vi "Change Boolean Image.vi"(6 "Mouse Position":T1, 7 "User VI Ref":refnum<vi>, 8 "Is Multi-select?":bool, 9 "Remaining Items":refnum<vi>[](array[refnum]), 10 "Affected Items":cluster{"Controls":refnum<vi>[]}, 11 "Menu Refnum":refnum<k9>) -> (3 "Menu Items To Add":T2[](array[typedef]))   [LabVIEW 2021]
doc: "This implementation of the right click menu VI will set the \"Boolean Type\" for a given Boolean control(s) for a VI. It will categorize the type of the button that is being used so that Theme-ing can be applied appropriately.\n\n<b>Original</b>: This VI is part of a plug-in for modifying the LabVIEW shortcut menus. This is the builder VI which is called when the shortcut menu is built. It tells LabVIEW which shortcut menu items to add to the menu."
uses:
  <resource>/plugins/PopupMenus/support/Shortcut Menu Item Definition.ctl
  <resource>/plugins/PopupMenus/support/Transaction Control.ctl
  <resource>/plugins/PopupMenus/support/Position In Menu.ctl
  <resource>/plugins/PopupMenus/support/Relative Position.ctl
  <resource>/plugins/PopupMenus/support/Checkmark Status.ctl
  <resource>/plugins/PopupMenus/support/Enabled Menu Item Status.ctl
  <vilib>/Utility/miscctls.llb/LVPositionTypeDef.ctl
panel:
  # "Rules a popup plug-in must follow:\n* This VI's file name must match the file name of the LLB -- only the file extensions should be different.\n* This VI must have debugging disabled or it will be ignored as a plug-in.\n* For all menu items, \"tag suffix + file name of this VI\" must be less than 240 characters.\n* You can disconnect the \"Affected Items\" from the typedef to make the plug-in load faster. The typedef is only there to assist you in keeping this VI and the execution VI using to the same type.\n* All controls on this panel except \"Affected Items\" are locked to prevent accidental edits. Do not change the types or the names of controls other than the elements inside the \"Affected Items\" cluster.\n* See Context Help for more information on the individual controls."
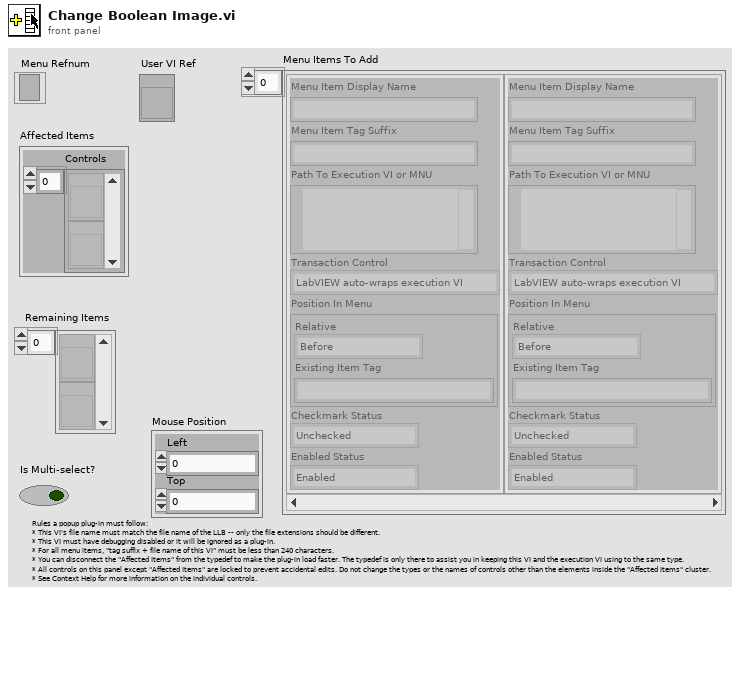
[diagram p1: front panel]
types:
  T1 = typedef "LVPositionTypeDef.ctl" = cluster{"Left":i32, "Top":i32}
  T2 = typedef "Shortcut Menu Item Definition.ctl" = cluster{"Menu Item Display Name":string, "Menu Item Tag Suffix":string, "Path To Execution VI or MNU":path, "Transaction Control":T3, "Position In Menu":T4, "Checkmark Status":T6, "Enabled Status":T7}
  T3 = typedef "Transaction Control.ctl" = enum8{"LabVIEW auto-wraps execution VI", "Execution VI will define if needed"}
  T4 = typedef "Position In Menu.ctl" = cluster{"Relative":T5, "Existing Item Tag":string}
  T5 = typedef "Relative Position.ctl" = enum8{"Before", "Instead of", "After", "Into Submenu"}
  T6 = typedef "Checkmark Status.ctl" = enum8{"Unchecked", "Checked"}
  T7 = typedef "Enabled Menu Item Status.ctl" = enum8{"Enabled", "Disabled"}
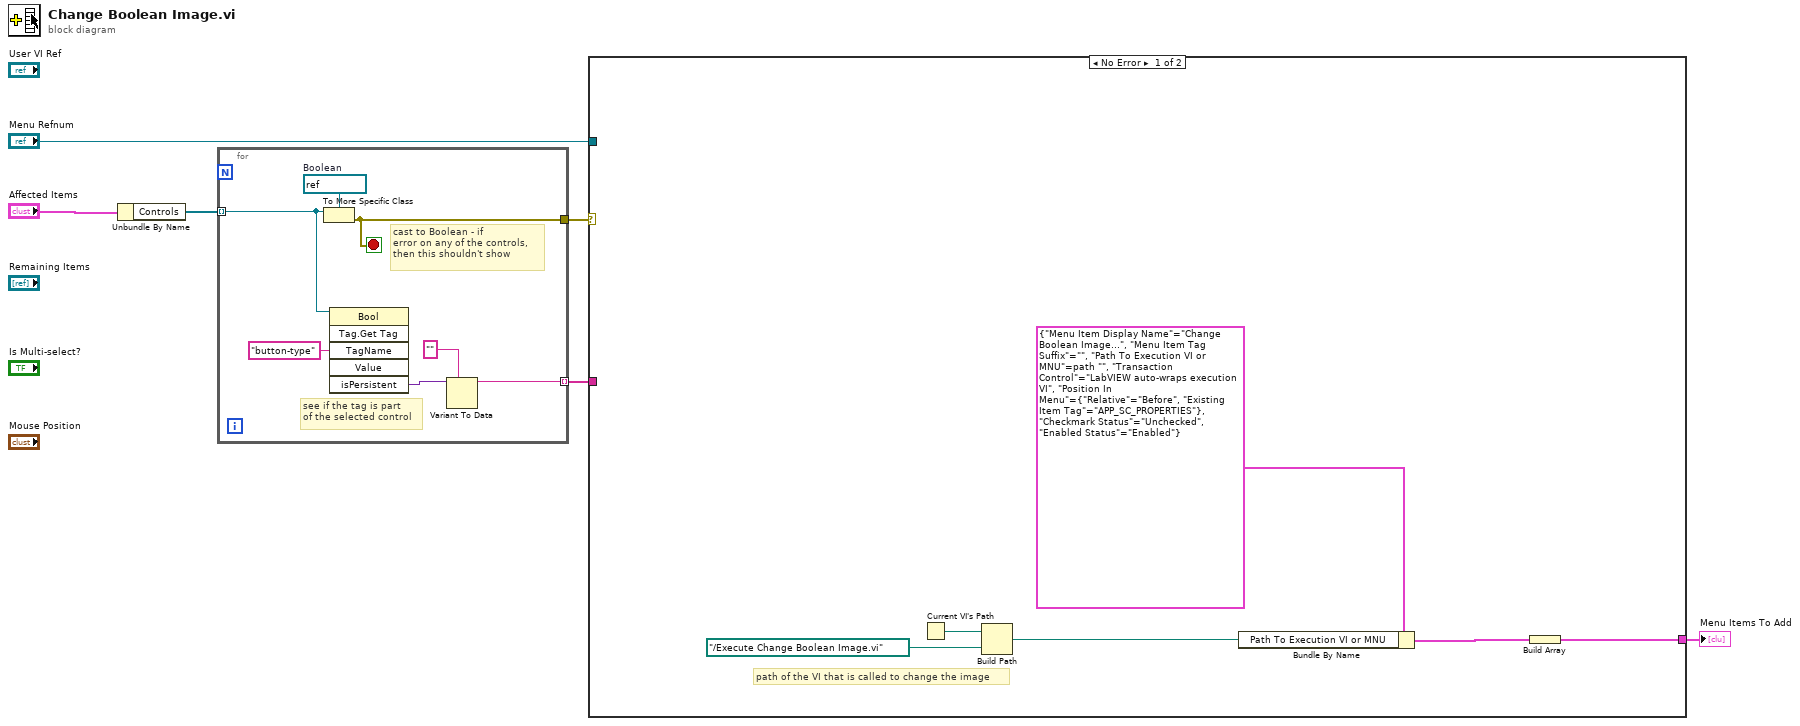
[diagram p0: block diagram]
diagram:
  n1 = Unbundle By Name("Affected Items") -> ("Controls"=w4:refnum<vi>[])
  n2 = for {
    tunnel: w4 -> [w7] mode=indexing
    tunnel: [w12] -> w3
    tunnel: [w8] -> w1 mode=indexing
    stop <- w12 stop-if-true
    w13 = refnum<vi> refnum  # Boolean
    # "cast to Boolean - if\nerror on any of the controls, \nthen this shouldn't show"
    # "see if the tag is part \nof the selected control"
    n3 = To More Specific Class(target class=w13, reference=w7) -> (error out=w12:errorcluster)  [unwired: 1 in, 1 out]
    n4 = invoke class="Bool" method="Tag.Get Tag"(reference=w7, "TagName"="button-type" ("Tag Name")) -> ("isPersistent"=w10:variant)  [unwired: 4 in, 5 out]
    n5 = Variant To Data(type="", Variant=w10) -> (data=w8:string)  [unwired: 1 in, 1 out]
  }
  n6 = case shown="No Error" w3 {
    tunnel: "Menu Refnum" -> [_ _]
    tunnel: [w14 _] -> w2
    tunnel: w1 -> [_ _]
    frame No Error {
      # "path of the VI that is called to change the image"
      n7 = Current VI's Path() -> (path=w18:path)
      n8 = Build Path(base path=w18, name or relative path=path "../Execute Change Boolean Image.vi" ("execute path")) -> (appended path=w16:path)
      n9 = Bundle By Name(cluster=T2 {"Menu Item Display Name"="Change Boolean Image...", "Menu Item Tag Suffix"="", "Path To Execution VI or MNU"=path "", "Transaction Control"=enum."LabVIEW auto-wraps execution VI", "Position In Menu"={"Relative"=enum."Before", "Existing Item Tag"="APP_SC_PROPERTIES"}, "Checkmark Status"=enum."Unchecked", "Enabled Status"=enum."Enabled"} ("Cluster"), "Path To Execution VI or MNU"=w16) -> (w15:T2)
      n10 = Build Array(w15) -> (w14:T2[])
    }
    frame Error {
    }
  }
  "Menu Items To Add" <- w2
